vi "Ox_ACFrontPanel_2Channel_ITC503_LKS370_4SRS830.vi"() -> ()   [LabVIEW 2014]
uses:
  <vilib>/Utility/file.llb/Write To Spreadsheet File (DBL).vi
  Lake Shore Cryotronics 370/Lake Shore Cryotronics 370.lvlib
panel:
  in  "Abort!":bool
  out "Timestamp":dbl format="%#_13g"
  in  "Tab Control":T1(tab)
  in  "Oxford Sweep Program":T2(array[cluster]) {"Hold Time For Stage" min=0.0 max=1339.9 step=0.1 format="%.2f"; "Sweep Time for Stage" min=0.0 max=1339.9 step=0.1 format="%.2f"; "Set Point" format="%.2f"}
  in  "LKS370":refnum<visa-resource-name>
  in  "SampleName":string
  in  "OxfordITC503s":refnum<visa-resource-name>
  in  "error in (no error)":errorcluster
  in  "SRS 3":refnum<visa-resource-name>
  in  "SRS 4":refnum<visa-resource-name>
  in  "SRS 2":refnum<visa-resource-name>
  in  "SRS 1":refnum<visa-resource-name>
  out "XY Graph 5":cluster{dbl, dbl}[](graph) caption="SRS1"
  out "XY Graph 6":cluster{dbl, dbl}[](graph) caption="SRS1"
  out "XY Graph 7":cluster{dbl, dbl}[](graph) caption="SRS1X"
  out "XY Graph 4":cluster{dbl, dbl}[](graph) caption="SRS1Y"
  out "XY Graph 9":cluster{dbl, dbl}[](graph) caption="SRS2 X"
  out "XY Graph 8":cluster{dbl, dbl}[](graph) caption="SRS2Y"
  out "XY Graph 11":cluster{dbl, dbl}[](graph) caption="SRS3X"
  out "XY Graph 12":cluster{dbl, dbl}[](graph) caption="SRS4Y"
  out "XY Graph 13":cluster{dbl, dbl}[](graph) caption="SRS4X"
  out "XY Graph 10":cluster{dbl, dbl}[](graph) caption="SRS3Y"
  out "Data is being stored here":string
  # "RealTime Data"
  # "Thermometry"
  # "INSTRUMENT ADDRESSES"
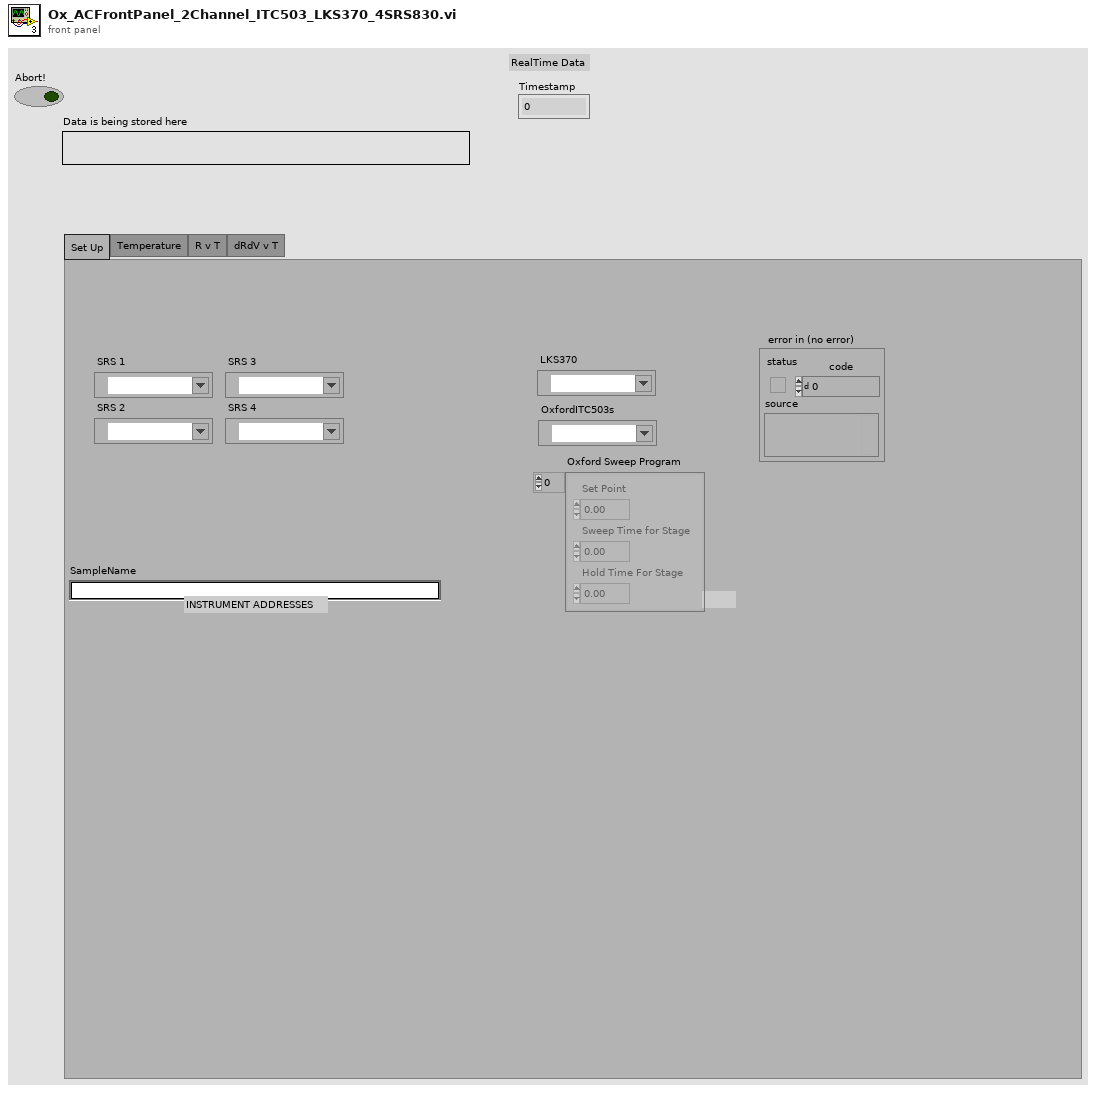
[diagram p1: front panel]
types:
  T1 = enum32{"Set Up", "Temperature", "R v T", "dRdV v T"}
  T2 = cluster{"Set Point":dbl, "Sweep Time for Stage":dbl, "Hold Time For Stage":dbl}[]
  T3 = cluster{"Elapsed Time (s)":dbl, "Kelvin Reading":dbl}
  T4 = cluster{"Elapsed Time (s)":dbl, "Kelvin Reading":dbl}[]
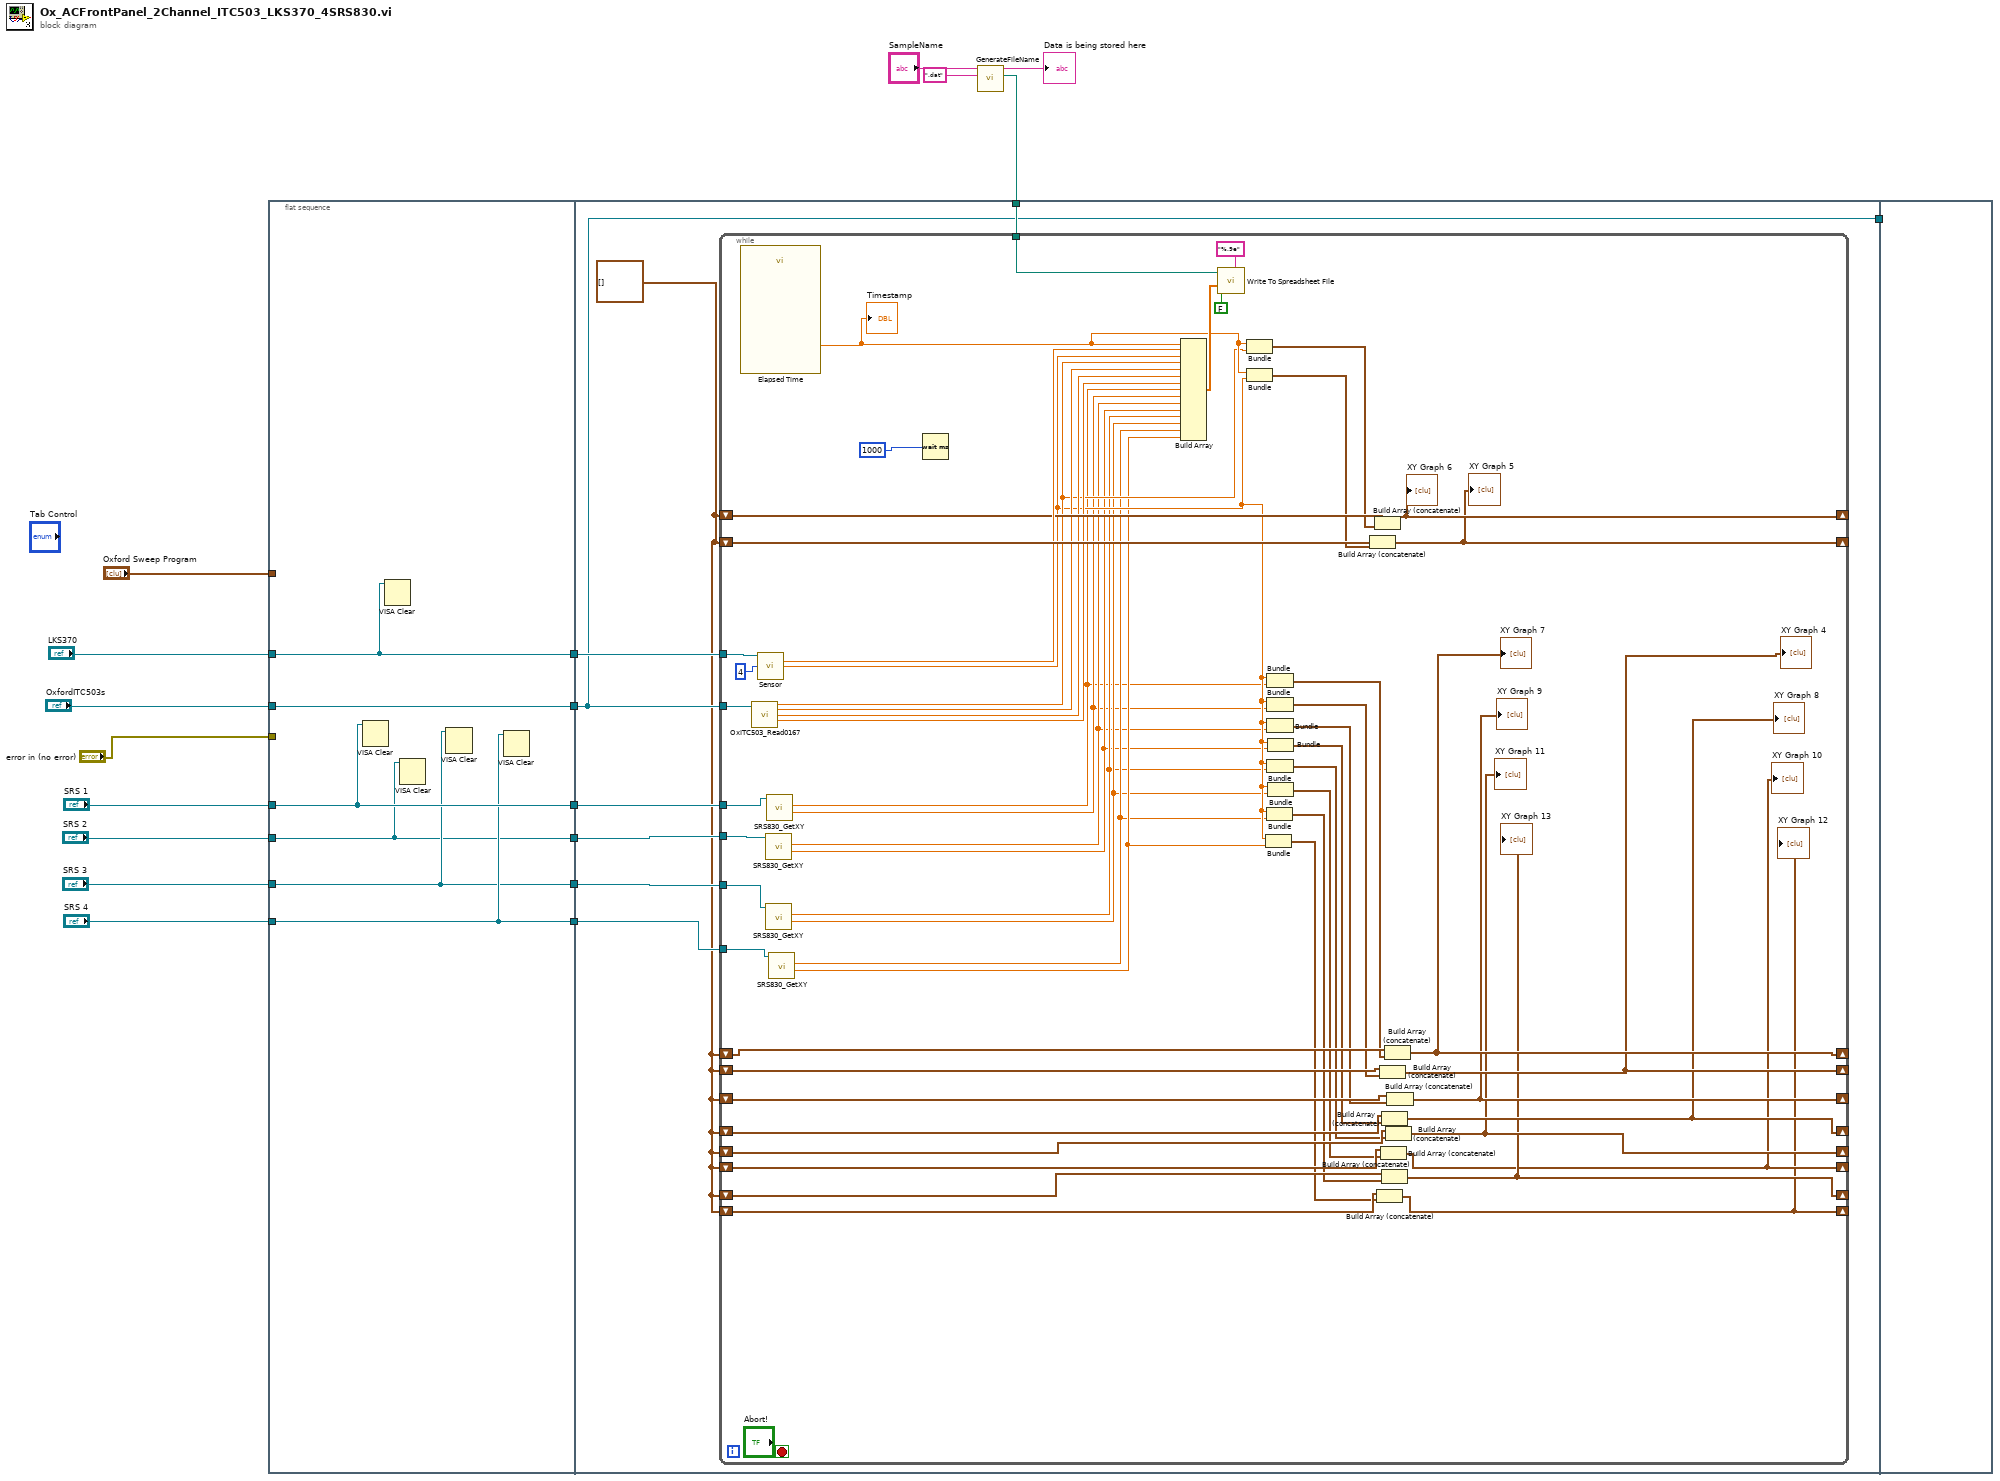
[diagram p0: block diagram]
diagram:
  n1 = flat-sequence {
    tunnel: "LKS370" -> [w20]
    tunnel: [w20] -> w15
    tunnel: [w25] -> w13
    tunnel: "OxfordITC503s" -> [w25]
    tunnel: "error in (no error)" -> [_]
    tunnel: "Oxford Sweep Program" -> [_]
    tunnel: [w24] -> w8
    tunnel: "SRS 1" -> [w24]
    tunnel: [w21] -> w6
    tunnel: "SRS 2" -> [w21]
    tunnel: [w22] -> w4
    tunnel: "SRS 3" -> [w22]
    tunnel: [w23] -> w2
    tunnel: "SRS 4" -> [w23]
    tunnel: w15 -> [w33]
    tunnel: w14 -> [w32]
    tunnel: w13 -> [w31]
    tunnel: [w31] -> w11
    tunnel: w8 -> [w30]
    tunnel: w6 -> [w29]
    tunnel: w4 -> [w28]
    tunnel: w2 -> [w27]
    tunnel: w11 -> [_]
    frame #0 {
      n2 = VISA Clear(VISA resource name=w24) -> ()  [unwired: 1 in, 2 out]
      n3 = VISA Clear(VISA resource name=w20) -> ()  [unwired: 1 in, 2 out]
      n4 = VISA Clear(VISA resource name=w21) -> ()  [unwired: 1 in, 2 out]
      n5 = VISA Clear(VISA resource name=w22) -> ()  [unwired: 1 in, 2 out]
      n6 = VISA Clear(VISA resource name=w23) -> ()  [unwired: 1 in, 2 out]
    }
    frame #1 {
      w26 = cluster{"T1":dbl, "Elapsed Time (s)":dbl}[] []
      n7 = while {
        tunnel: w33 -> [w86]
        tunnel: w32 -> [w87]
        tunnel: w31 -> [w78]
        shift-right: [w71] -> _
        shift-left: w26 -> [w85]
        shift-right: [w80] -> _
        shift-left: w26 -> [w81]
        tunnel: w30 -> [w70]
        tunnel: w29 -> [w69]
        tunnel: w28 -> [w68]
        tunnel: w27 -> [w67]
        shift-right: [w41] -> _
        shift-left: w26 -> [w66]
        shift-right: [w39] -> _
        shift-left: w26 -> [w64]
        shift-right: [w40] -> _
        shift-left: w26 -> [w65]
        shift-right: [w38] -> _
        shift-left: w26 -> [w63]
        shift-right: [w37] -> _
        shift-left: w26 -> [w62]
        shift-right: [w35] -> _
        shift-left: w26 -> [w61]
        shift-right: [w36] -> _
        shift-left: w26 -> [w60]
        shift-right: [w34] -> _
        shift-left: w26 -> [w59]
        stop <- "Abort!" stop-if-true
        n8 = call "Elapsed Time"() -> ("Elapsed Time (s)"=w79:dbl)  [unwired: 12 in, 7 out]
        "Timestamp" <- w79
        n9 = call "OxITC503_Read0167.vi"("VISA session 2"=w78) -> ("Temp"=w74:dbl, "SetPoint"=w77:dbl, "Heater\nOutput"=w76:dbl, "GasFlow"=w75:dbl)  [unwired: 9 in, 2 out]
        n10 = call "Sensor.vi"("VISA resource name"=w86, "Channel (1)"=4) -> ("Resistance Reading"=w83:dbl, "Kelvin Reading"=w58:dbl)  [unwired: 9 in, 3 out]
        n11 = call "SRS830_GetXY.vi"("SRS 830"=w69) -> ("Y"=w53:dbl, "X"=w52:dbl)  [unwired: 7 in, 2 out]
        n12 = call "SRS830_GetXY.vi"("SRS 830"=w68) -> ("Y"=w55:dbl, "X"=w54:dbl)  [unwired: 7 in, 2 out]
        n13 = call "SRS830_GetXY.vi"("SRS 830"=w70) -> ("Y"=w51:dbl, "X"=w50:dbl)  [unwired: 7 in, 2 out]
        n14 = call "SRS830_GetXY.vi"("SRS 830"=w67) -> ("Y"=w57:dbl, "X"=w56:dbl)  [unwired: 7 in, 2 out]
        n15 = Wait (ms)(milliseconds to wait=1000) -> ()  [unwired: 1 out]
        n16 = Build Array(w79, w83, w58, w74, w77, w76, w75, w50, w51, w52, w53, w54, w55, w56, w57) -> (w90:dbl[])
        n17 = call-poly <vilib>:"Write To Spreadsheet File.vi"("format (%.3f)"="%.9e", "append to file? (new file:F)"=FALSE, "1D data"=w90, "file path (dialog if empty)"=w87) -> ()  [unwired: 4 in, 1 out]
        n18 = Bundle("Elapsed Time (s)"=w79, "Temp"=w74) -> (w73:cluster{"Elapsed Time (s)":dbl, "Temp":dbl})  [unwired: 1 in]
        n19 = Bundle("Elapsed Time (s)"=w79, "Kelvin Reading"=w58) -> (w72:T3)  [unwired: 1 in]
        n20 = Bundle("Kelvin Reading"=w58, "Y"=w57) -> (w42:cluster{"Kelvin Reading":dbl, "Y":dbl})  [unwired: 1 in]
        n21 = Bundle("Kelvin Reading"=w58, "X"=w56) -> (w43:cluster{"Kelvin Reading":dbl, "X":dbl})  [unwired: 1 in]
        n22 = Bundle("Kelvin Reading"=w58, "X"=w50) -> (w49:cluster{"Kelvin Reading":dbl, "X":dbl})  [unwired: 1 in]
        n23 = Bundle("Kelvin Reading"=w58, "Y"=w51) -> (w48:cluster{"Kelvin Reading":dbl, "Y":dbl})  [unwired: 1 in]
        n24 = Bundle("Kelvin Reading"=w58, "X"=w52) -> (w47:cluster{"Kelvin Reading":dbl, "X":dbl})  [unwired: 1 in]
        n25 = Bundle("Kelvin Reading"=w58, "X"=w54) -> (w44:cluster{"Kelvin Reading":dbl, "X":dbl})  [unwired: 1 in]
        n26 = Bundle("Kelvin Reading"=w58, "Y"=w53) -> (w46:cluster{"Kelvin Reading":dbl, "Y":dbl})  [unwired: 1 in]
        n27 = Bundle("Kelvin Reading"=w58, "Y"=w55) -> (w45:cluster{"Kelvin Reading":dbl, "Y":dbl})  [unwired: 1 in]
        n28 = Build Array (concatenate)(w85, w72) -> (w71:T4)
        "XY Graph 5" <- w71
        n29 = Build Array (concatenate)(w81, w73) -> (w80:cluster{"Elapsed Time (s)":dbl, "Temp":dbl}[])
        "XY Graph 6" <- w80
        n30 = Build Array (concatenate)(w59, w42) -> (w34:cluster{"Kelvin Reading":dbl, "Y":dbl}[])
        "XY Graph 12" <- w34
        n31 = Build Array (concatenate)(w65, w48) -> (w40:cluster{"Kelvin Reading":dbl, "Y":dbl}[])
        "XY Graph 4" <- w40
        n32 = Build Array (concatenate)(w61, w45) -> (w35:cluster{"Kelvin Reading":dbl, "Y":dbl}[])
        "XY Graph 10" <- w35
        n33 = Build Array (concatenate)(w63, w46) -> (w38:cluster{"Kelvin Reading":dbl, "Y":dbl}[])
        "XY Graph 8" <- w38
        n34 = Build Array (concatenate)(w60, w43) -> (w36:cluster{"Kelvin Reading":dbl, "X":dbl}[])
        "XY Graph 13" <- w36
        n35 = Build Array (concatenate)(w66, w49) -> (w41:cluster{"Kelvin Reading":dbl, "X":dbl}[])
        "XY Graph 7" <- w41
        n36 = Build Array (concatenate)(w62, w44) -> (w37:cluster{"Kelvin Reading":dbl, "X":dbl}[])
        "XY Graph 11" <- w37
        n37 = Build Array (concatenate)(w64, w47) -> (w39:cluster{"Kelvin Reading":dbl, "X":dbl}[])
        "XY Graph 9" <- w39
      }
    }
    frame #2 {
    }
  }
  n38 = call "GenerateFileName.vi"("FileExtension"=".dat", "SampleName"="SampleName") -> ("FilePathOut"=w14:path, "FolderNameString"=→"Data is being stored here":string)  [unwired: 3 in, 1 out]
